vi "Get Valid Properties.vi"(8 "error in (no error)":errorcluster, 11 "Gate in":refnum<class "Gate.lvclass">) -> (0 "error out":errorcluster, 2 "Properties":string[](array[string]), 3 "Gate out":refnum<class "Gate.lvclass">)   [LabVIEW 2020, in "Gate.lvclass"]
uses:
  Gate.lvclass
  Gate.lvclass/Gate.ctl
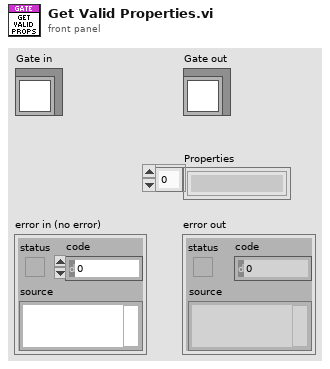
[diagram p1: front panel]
types:
  T1 = typedef "Gate.lvclass/Shape.ctl" = enum16{"OFF", "Rectangle", "Sine-squared", "Trapezoid"}
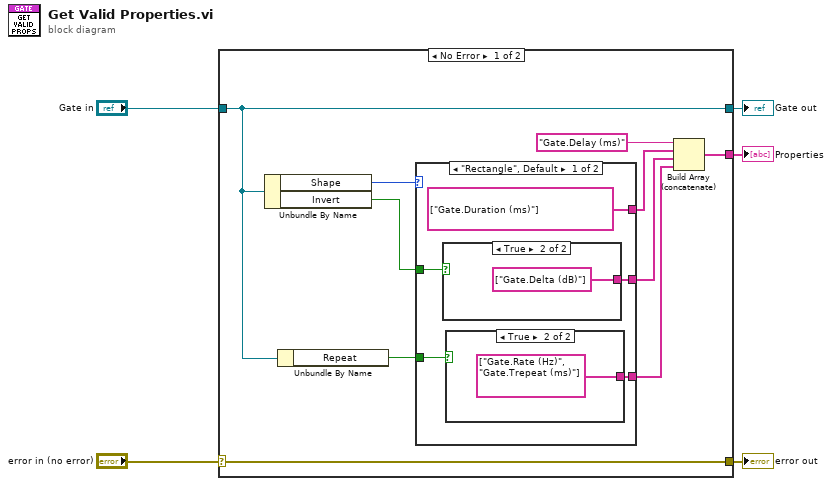
[diagram p0: block diagram]
diagram:
  n1 = case shown="No Error" "error in (no error)" {
    selector: "error in (no error)" -> [w15 w24]
    tunnel: [w15 w24] -> w4
    tunnel: [w8 w23] -> w2
    tunnel: "Gate in" -> [w8 w23]
    tunnel: [w11 _] -> w1
    frame No Error {
      n2 = Unbundle By Name(w8) -> ("Shape"=w12:T1, "Invert"=w10:bool)
      n3 = Unbundle By Name(w8) -> ("Repeat"=w7:bool)
      n4 = case shown="\"Rectangle\", Default" w12 {
        tunnel: [string[] ["Gate.Duration (ms)"] _] -> w13
        tunnel: w10 -> [w19 _]
        tunnel: [w18 _] -> w9
        tunnel: w7 -> [w17 _]
        tunnel: [w16 _] -> w6
        frame "Rectangle", Default {
          n5 = case shown="True" w19 {
            tunnel: [_ string[] ["Gate.Delta (dB)"]] -> w18
            frame False {
            }
            frame True {
            }
          }
          n6 = case shown="True" w17 {
            tunnel: [_ string[] ["Gate.Rate (Hz)", "Gate.Trepeat (ms)"]] -> w16
            frame False {
            }
            frame True {
            }
          }
        }
        frame "OFF" {
        }
      }
      n7 = Build Array (concatenate)("Gate.Delay (ms)", w13, w9, w6) -> (w11:string[])
    }
    frame Error {
    }
  }
  "error out" <- w4
  "Gate out" <- w2
  "Properties" <- w1
